vi "Determine Warnings.vi"(6 "최대 풍속":dbl, 7 "현재 풍속":dbl, 8 "에러 입력(에러 없음)":errorcluster, 9 "최저 온도":dbl, 10 "최고 온도":dbl, 11 "현재 온도":dbl) -> (0 "에러 없음":errorcluster caption="에러 출력", 1 "경고?":bool, 2 "경고 텍스트":string)   [LabVIEW 2010]
uses:
  Det Warnings.ctl
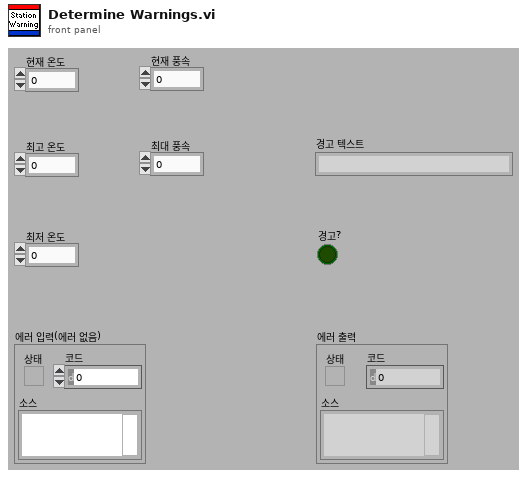
[diagram p1: front panel]
types:
  T1 = typedef "Det Warnings.ctl" = enum16{"열사병", "동상", "강풍", "경고 생성", "에러 확인"}
  T2 = cluster{"현재 온도":dbl, "최고 온도":dbl, "최저 온도":dbl, "현재 풍속":dbl, "최대 풍속":dbl}
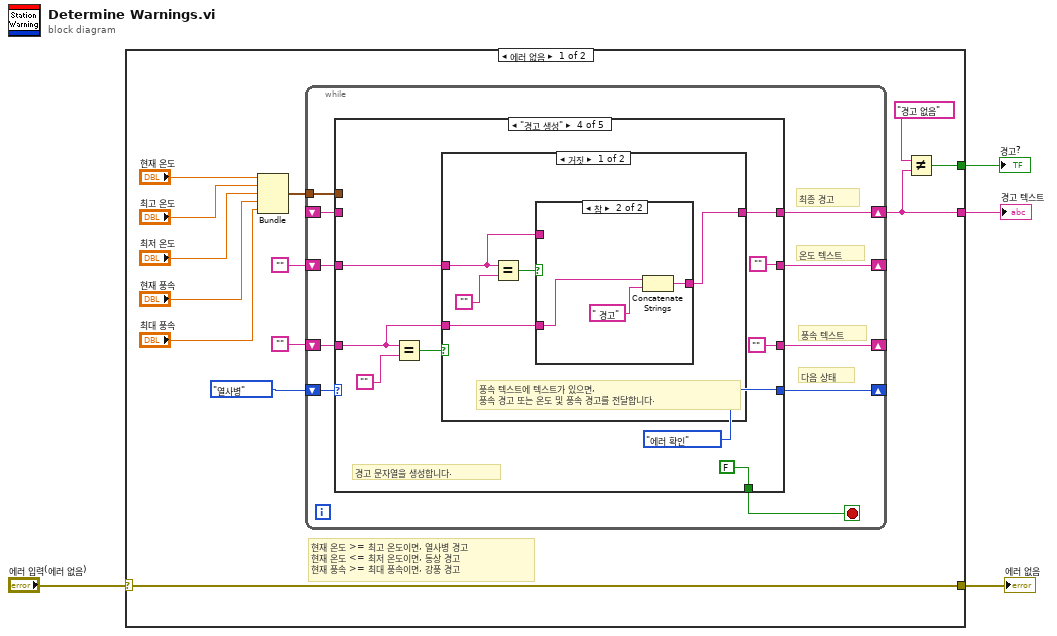
[diagram p0: block diagram]
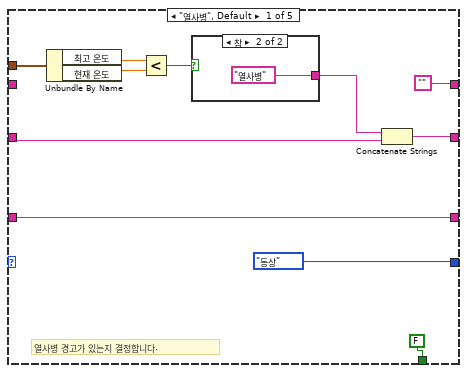
[diagram p2: hidden frame]
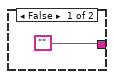
[diagram p3: hidden frame]
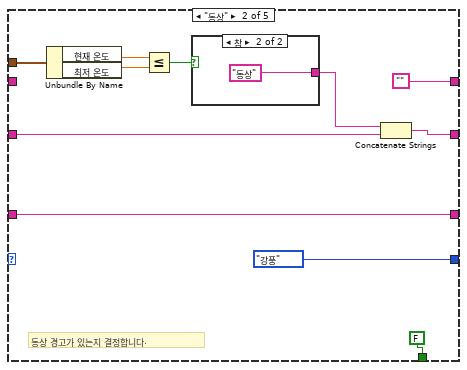
[diagram p4: hidden frame]
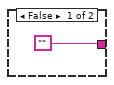
[diagram p5: hidden frame]
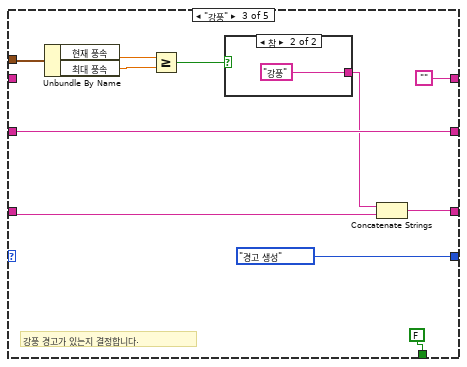
[diagram p6: hidden frame]
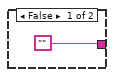
[diagram p7: hidden frame]
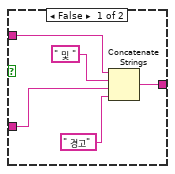
[diagram p8: hidden frame]
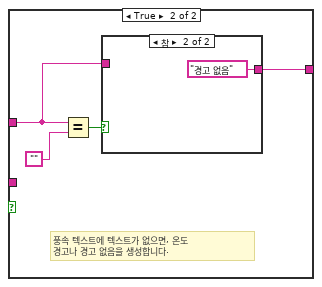
[diagram p9: hidden frame]
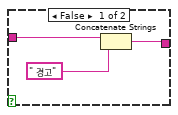
[diagram p10: hidden frame]
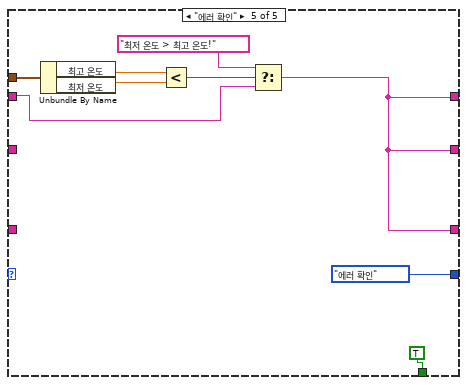
[diagram p11: hidden frame]
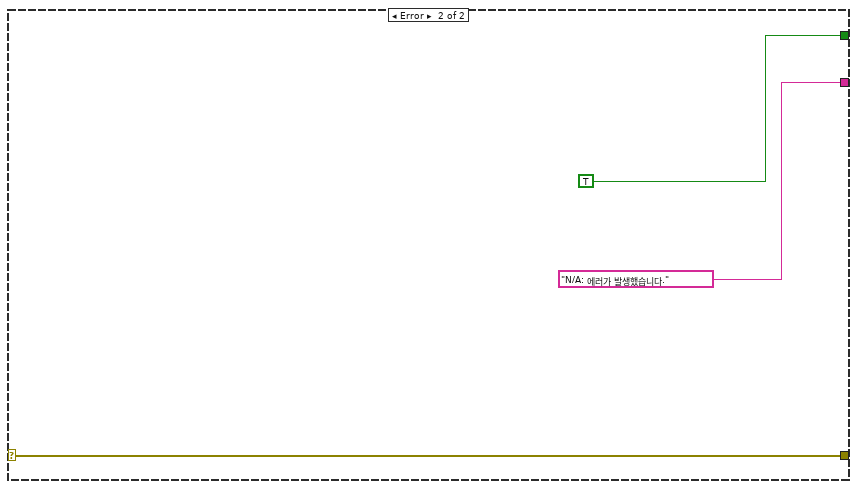
[diagram p12: hidden frame]
diagram:
  n1 = case shown="에러 없음" "에러 입력(에러 없음)" {
    selector: "에러 입력(에러 없음)" -> [w16 w108]
    tunnel: [w16 w108] -> w3
    tunnel: [w17 TRUE] -> w2
    tunnel: [w6 "N/A: 에러가 발생했습니다." ("f")] -> w1
    frame No Error {
      # "현재 온도 >= 최고 온도이면, 열사병 경고\n현재 온도 <= 최저 온도이면, 동상 경고\n현재 풍속 >= 최대 풍속이면, 강풍 경고"
      n2 = Bundle("현재 온도"="현재 온도", "최고 온도"="최고 온도", "최저 온도"="최저 온도", "현재 풍속"="현재 풍속", "최대 풍속"="최대 풍속") -> (w9:T2)  [unwired: 1 in]
      n3 = while {
        tunnel: w9 -> [w24]
        shift-right: [w23] -> _
        shift-left: Det_Warnings."열사병" ("Enum") -> [w27]
        shift-right: [w26] -> _
        shift-left: "" -> [w22]
        shift-right: [w25] -> _
        shift-left: "" -> [w21]
        shift-right: [w20] -> w6
        shift-left: _ -> [w18]
        stop <- w19 stop-if-true
        # "최종 경고"
        # "다음 상태"
        # "풍속 텍스트"
        # "온도 텍스트"
        n4 = case shown="\"경고 생성\"" w27 {
          tunnel: [w30 w46 w58 "" w99] -> w25
          tunnel: [w33 w45 w59 "" w99] -> w26
          tunnel: w24 -> [w37 w51 w64 _ w105]
          tunnel: [Det_Warnings."동상" ("Enum") Det_Warnings."강풍" ("Enum") Det_Warnings."경고 생성" ("Enum") Det_Warnings."에러 확인" ("Enum") Det_Warnings."에러 확인" ("Enum")] -> w23
          tunnel: w22 -> [w32 w43 w59 w75 _]
          tunnel: w21 -> [w30 w46 w56 w72 _]
          tunnel: ["" "" "" w71 w99] -> w20
          tunnel: [FALSE FALSE FALSE FALSE TRUE] -> w19
          tunnel: w18 -> [_ _ _ _ w101]
          frame "열사병", Default {
            # "열사병 경고가 있는지 결정합니다."
            n5 = Unbundle By Name(w37) -> ("최고 온도"=w36:dbl, "현재 온도"=w35:dbl)
            n6 = Less?(x=w36, y=w35) -> (x < y?=w38:bool)
            n7 = case shown="참" w38 {
              tunnel: ["" "열사병"] -> w31
              frame False {
              }
              frame True {
              }
            }
            n8 = Concatenate Strings(w31, w32) -> (w33:string)
          }
          frame "동상" {
            # "동상 경고가 있는지 결정합니다."
            n9 = Unbundle By Name(w51) -> ("현재 온도"=w49:dbl, "최저 온도"=w48:dbl)
            n10 = Less Or Equal?(x=w49, y=w48) -> (x <= y?=w50:bool)
            n11 = case shown="참" w50 {
              tunnel: ["" "동상"] -> w44
              frame False {
              }
              frame True {
              }
            }
            n12 = Concatenate Strings(w44, w43) -> (w45:string)
          }
          frame "강풍" {
            # "강풍 경고가 있는지 결정합니다."
            n13 = Unbundle By Name(w64) -> ("현재 풍속"=w63:dbl, "최대 풍속"=w62:dbl)
            n14 = Greater Or Equal?(x=w63, y=w62) -> (x >= y?=w61:bool)
            n15 = case shown="참" w61 {
              tunnel: ["" "강풍"] -> w57
              frame False {
              }
              frame True {
              }
            }
            n16 = Concatenate Strings(w57, w56) -> (w58:string)
          }
          frame "경고 생성" {
            # "경고 문자열을 생성합니다."
            n17 = Equal?(x=w72, y="") -> (x = y?=w73:bool)
            n18 = case shown="거짓" w73 {
              tunnel: [w78 w92] -> w71
              tunnel: w75 -> [w76 w89]
              tunnel: w72 -> [w77 _]
              frame False {
                # "풍속 텍스트에 텍스트가 있으면,\n풍속 경고 또는 온도 및 풍속 경고를 전달합니다."
                n19 = Equal?(x=w76, y="") -> (x = y?=w79:bool)
                n20 = case shown="참" w79 {
                  tunnel: [w83 w87] -> w78
                  tunnel: w77 -> [w82 w86]
                  tunnel: w76 -> [w81 _]
                  frame False {
                    n21 = Concatenate Strings(w81, " 및 " ("string"), w82, " 경고" ("string")) -> (w83:string)
                  }
                  frame True {
                    n22 = Concatenate Strings(w86, " 경고" ("string")) -> (w87:string)
                  }
                }
              }
              frame True {
                # "풍속 텍스트에 텍스트가 없으면, 온도\n경고나 경고 없음을 생성합니다."
                n23 = Equal?(x=w89, y="") -> (x = y?=w90:bool)
                n24 = case shown="참" w90 {
                  tunnel: [w95 "경고 없음"] -> w92
                  tunnel: w89 -> [w94 _]
                  frame False {
                    n25 = Concatenate Strings(w94, " 경고") -> (w95:string)
                  }
                  frame True {
                  }
                }
              }
            }
          }
          frame "에러 확인" {
            n26 = Unbundle By Name(w105) -> ("최고 온도"=w104:dbl, "최저 온도"=w103:dbl)
            n27 = Less?(x=w104, y=w103) -> (x < y?=w102:bool)
            n28 = Select(t="최저 온도 > 최고 온도!", s=w102, f=w101) -> (s? t:f=w99:string)
          }
        }
      }
      n29 = Not Equal?(x="경고 없음", y=w6) -> (x != y?=w17:bool)
    }
    frame Error {
    }
  }
  "에러 없음" <- w3
  "경고 텍스트" <- w1
  "경고?" <- w2
